vi "ExSubCreateImage.vi"(2 "error in (no error)":errorcluster, 3 "Pulser Handle":u32, 4 "Camera Handle":u32) -> (0 "error out":errorcluster, 1 "Handles Out":T1)   [LabVIEW 2010]
panel:
  # "ExSubCreateFileDisplay:\nThis is a SubVI that creates a file, display and image \nobjects and returns the handles bundled in a cluster \nthat includes a pulser and camera handle"
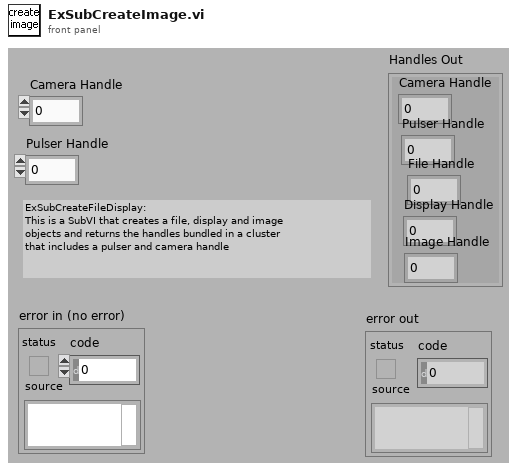
[diagram p1: front panel]
types:
  T1 = cluster{"Camera Handle":u32, "Pulser Handle":u32, "File Handle":u32, "Display Handle":u32, "Image Handle":u32}
  T2 = cluster{"Camera Handle":u32, "Pulser Handle":u32, i32, i32, "Image Handle":u32}
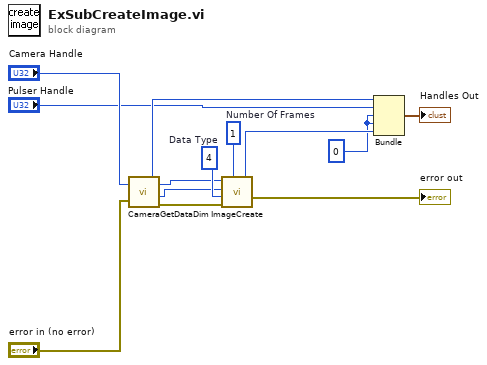
[diagram p0: block diagram]
diagram:
  w3 = 0
  w6 = u32 1  # Number Of Frames
  w7 = u32 4  # Data Type
  n1 = call <userlib>:"CameraGetDataDim.vi"("Camera Handle"="Camera Handle", "error in"="error in (no error)") -> ("Camera Handle"=w10:u32, "Xdim"=w4:u32, "Ydim"=w5:u32, "error out"=w13:errorcluster)
  n2 = call <userlib>:"ImageCreate.vi"("X dimension"=w4, "Y dimension"=w5, "Data Type"=w7, "error in"=w13, "Number Of Frames"=w6) -> ("Image Handle"=w8:u32, "error out"=→"error out":errorcluster)
  n3 = Bundle("Camera Handle"=w10, "Pulser Handle"="Pulser Handle", w3, w3, "Image Handle"=w8) -> (→"Handles Out":T2)  [unwired: 1 in]
